vi "WriteSF_one.vi"(1 "connection ID in":refnum<k5>, 2 "Steering value":u8, 3 "Motor value":u8=100, 4 "destination ID":u16) -> (0 "connection ID out":refnum<k5>)   [LabVIEW 2010]
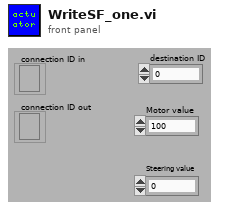
[diagram p1: front panel]
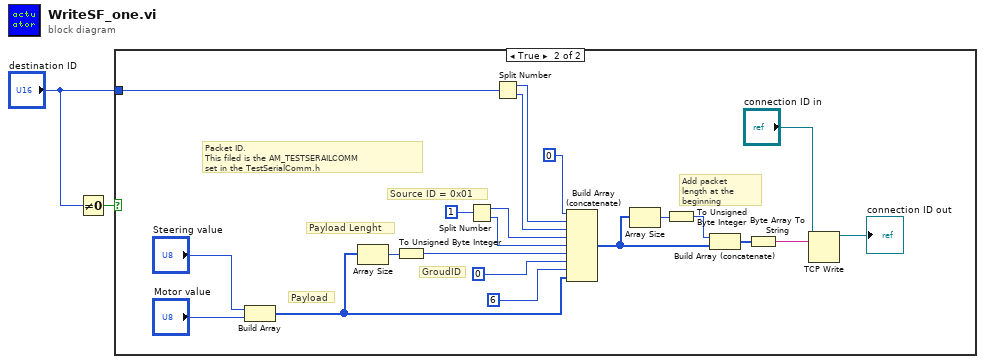
[diagram p0: block diagram]
diagram:
  n1 = Not Equal To 0?(x="destination ID") -> (x != 0?=w2:bool)
  n2 = case shown="True" w2 {
    tunnel: "destination ID" -> [_ w4]
    frame False {
    }
    frame True {
      # "Add packet\nlength at the\nbeginning"
      # "Payload"
      # "Packet ID.\nThis filed is the AM_TESTSERAILCOMM \nset in the TestSerialComm.h"
      # "GroudID"
      # "Payload Lenght"
      # "Source ID = 0x01"
      n3 = Build Array("Steering value", "Motor value") -> (w16:u8[])
      n4 = Array Size(array=w16) -> (size(s)=w15:i32)
      n5 = To Unsigned Byte Integer(number=w15) -> (unsigned 8bit integer=w14:u8)
      n6 = Split Number(x=u16 1 ("Actuator ID\nBlue")) -> (hi(x)=w8:u8, lo(x)=w7:u8)
      n7 = Split Number(x=w4) -> (hi(x)=w20:u8, lo(x)=w19:u8)
      n8 = Build Array (concatenate)(u8 0, w20, w19, w8, w7, w14, u8 0, u8 6, w16) -> (w12:u8[])
      n9 = Array Size(array=w12) -> (size(s)=w11:i32)
      n10 = To Unsigned Byte Integer(number=w11) -> (unsigned 8bit integer=w10:u8)
      n11 = Build Array (concatenate)(w10, w12) -> (w9:u8[])
      n12 = Byte Array To String(unsigned byte array=w9) -> (string=w13:string)
      n13 = TCP Write(connection ID="connection ID in", data in=w13) -> (connection ID out=→"connection ID out":refnum<k5>)  [unwired: 2 in, 2 out]
    }
  }
